vi "Volts to ADC.vi"(2 "maxValue":u16, 3 "value in Volt":dbl) -> (1 "ADC value":u16)   [LabVIEW 2016, in "pl1000.lvlib"]
doc: "Converts value in Volt to value in raw ADC counts.\n\n<b>maxValue</b> is the output of pl1000MaxValue.vi"
uses:
  pl1000.lvlib
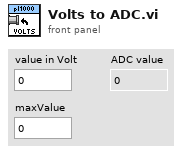
[diagram p1: front panel]
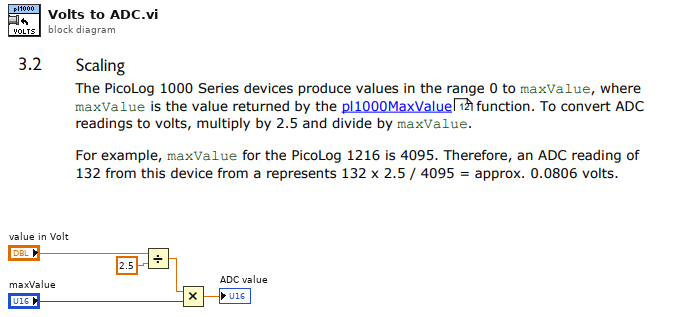
[diagram p0: block diagram]
diagram:
  n1 = Divide(x="value in Volt", y=2.5) -> (x/y=w3:dbl)
  n2 = Multiply(x=w3, y="maxValue") -> (x*y=→"ADC value":dbl)
